vi "Actor Core.vi"(8 "error in":errorcluster, 11 "Contador_Actor_Interface in":refnum<class "Contador_Actor_Interface.lvclass">) -> (0 "error out":errorcluster, 3 "Actor out":refnum<class "Actor.lvclass">)   [LabVIEW 2019, in "Contador_Actor_Interface.lvlib" / "Contador_Actor_Interface.lvclass"]
doc: "(<B>Filename</B>: Actor Framework.lvlib:Actor.lvclass:Actor Core.vi)\n\nReceives messages to the actor, reacts to them, and initiates any error handling that may shut the actor down.\n\nDescendant classes may override this VI to append parallel tasks for the actor to complete while it handles messages. Overrides use the Call Parent Method node."
uses:
  Contador_Actor_Interface.lvclass
  <vilib>/ActorFramework/Actor/Actor.lvclass
panel:
  in  "Save":bool
  in  "Path":path
  in  "Exit":bool
  in  "Stop":bool
  in  "Start":bool
  out "Boolean array":bool[](array[boolean])
  in  "Lim. Superior":u8
  in  "Lim. Inferior":u8
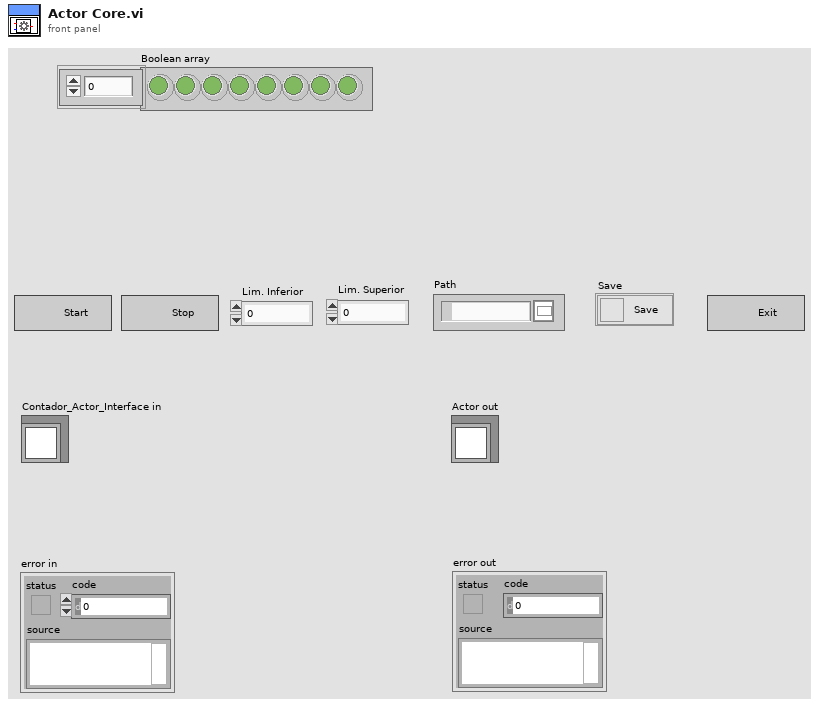
[diagram p1: front panel]
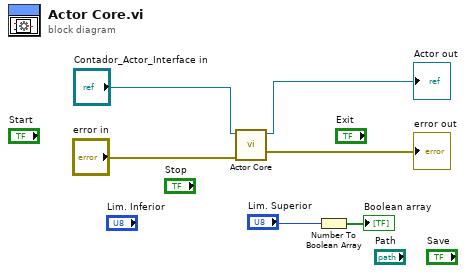
[diagram p0: block diagram]
diagram:
  n1 = call-parent "Actor Core.vi"("error in"="error in", "Actor in"="Contador_Actor_Interface in") -> ("error out"=→"error out":errorcluster, "Actor out"=→"Actor out":refnum<class "Actor.lvclass">)  [unwired: 8 in]
  n2 = Number To Boolean Array(number="Lim. Superior") -> (Boolean array=→"Boolean array":bool[])
